vi "WeirdData.vi"() -> ()   [LabVIEW 2011]
panel:
  out "size(s)":i32
  in  "Path:~\\syslogs\\FalconProcessed":path
  in  "ProcessedData":u8[](array[numeric])=array[44904 elements]
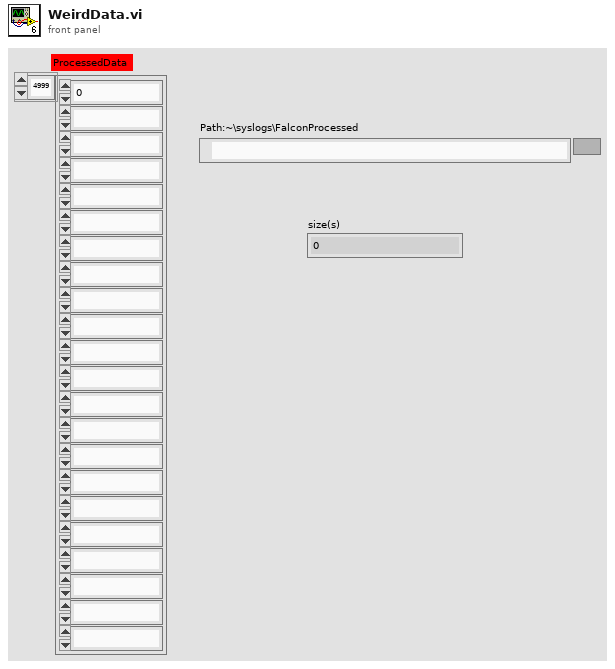
[diagram p1: front panel]
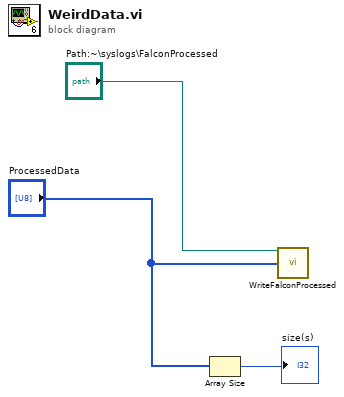
[diagram p0: block diagram]
diagram:
  n1 = Array Size(array="ProcessedData") -> (size(s)=→"size(s)":i32)
  n2 = call "WriteFalconProcessed.vi"("Path:~\\syslogs\\FalconProcessed"="Path:~\\syslogs\\FalconProcessed", "FalconProcessedData"="ProcessedData") -> ()  [unwired: 13 in, 1 out]
